vi "calConverToND.vi"(9 "O3 Flow, sccm (80)":dbl, 10 "flows, sccm":dbl[][](array[numeric]), 11 "[o3], ppb":dbl[][](array[numeric])) -> (3 "Array":dbl[](array[numeric]))   [LabVIEW 2011]
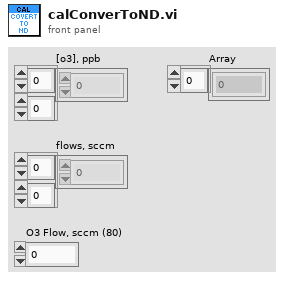
[diagram p1: front panel]
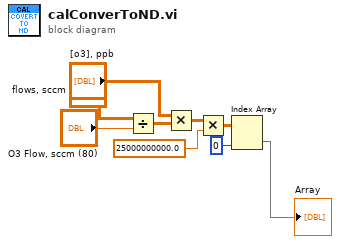
[diagram p0: block diagram]
diagram:
  n1 = Divide(x="flows, sccm", y="O3 Flow, sccm (80)") -> (x/y=w3:dbl[][])
  n2 = Multiply(x="[o3], ppb", y=w3) -> (x*y=w5:dbl[][])
  n3 = Multiply(x=w5, y=25000000000.0 ("simga-532")) -> (x*y=w7:dbl[][])
  n4 = Index Array(array=w7, index (col)=0 ("disabled index (col)")) -> (element=→"Array":dbl[])  [unwired: 1 in]
